vi "WiFi Receiver(FPGA).vi"() -> ()   [LabVIEW 2020]
doc: "Acquires data from the Rx ports and streams the data to the host while receiving data from the host and generating the resulting waveform at the Tx ports of the NI USRP 294x/295x device. Use this VI as a template for the Simple NI-USRP Streaming sample project."
uses:
  <instrlib>/_niInstr/Register Bus/v1/FPGA/Public/Read Cmd Data.ctl
  SubVIs/Stream Control State.ctl
  SubVIs/Rx Parameters 2945 2955.ctl
  Host/SubVIs/Start Trigger.ctl
  SubVIs/DDC Parameters 2945 2955.ctl
  <instrlib>/_niInstr/DSP/v1/Shared/Public/IQ Impairments.ctl
  <instrlib>/_niInstr/DSP/v1/Shared/Public/IQ Gain.ctl
  FPGA Bitfiles/Configuration Control.ctl
  <vilib>/Platform/TimedLoop/XDataNode/timing_clust.ctl
  <vilib>/Platform/TimedLoop/XDataNode/nitl_modes.ctl
  <vilib>/Platform/TimedLoop/XDataNode/wakeup.ctl
  SubVIs/Tx Parameters.ctl
  SubVIs/DUC Parameters.ctl
  <vilib>/rvi/Emulation/niFpgaSctlEmulationGetInTimedLoop.vi
  <vilib>/rvi/Emulation/niFpgaEmulationReportErrorSimple.vi
  <vilib>/rvi/Emulation/niFpgaGetClockAttributes.vi
  <vilib>/rvi/Emulation/niFpgaCriticalErrorInLSC.vi
  <vilib>/rvi/DataTransferAndStorage/Container/Common/niFpgaContainerExecOnDevCompGetState.vi
  <vilib>/rvi/Emulation/niFpgaEmulationIsFPGAContextNoSignature.vi
  <vilib>/rvi/errors/niFpgaSetErrorForExecOnDevCompSimple.vi
  <vilib>/rvi/eio/common/nirviEmuReportErrorAndStop.vi
  <vilib>/rvi/DataTransferAndStorage/Container/Common/niFpgaContainerGetUniqueNameForEmu.vi
  <vilib>/rvi/FIFO/Fifo_Resource/nirvififoEmulationSetSize.vi
  <vilib>/rvi/FIFO/Fifo_Resource/nirviFifoEmulationQueueMgr.vi
  <instcachedir>/0/nirviFifoEmulationQueueMgr_E5CAEC123FF24DC58D834DCA3CDAA9B5.lvgen/nirviFifoEmulationQueueMgr_E5CAEC123FF24DC58D834DCA3CDAA9B5_004.vi
  <vilib>/rvi/FIFO/Fifo_Resource/nirvififoEmulationDetermineInputValidOut.vi
  <vilib>/rvi/FIFO/Fifo_Resource/nirvififoEmulationCreateLock.vi
  <vilib>/rvi/Emulation/niFpgaProcessEmulError.vi
  <vilib>/rvi/FIFO/Fifo_Resource/nirvififoEmulationObtainLock.vi
  <vilib>/rvi/FIFO/Fifo_Resource/nirvififoEmulationReleaseLock.vi
  <vilib>/rvi/occurrence/nirviWaitOnOccurrenceBase.vi
  <vilib>/rvi/errors/nirviReportUnexpectedCaseInternalError.vi
  <vilib>/rvi/errors/nirviReportUnexpectedCaseInternalError (U32).vi
  <vilib>/Utility/error.llb/Clear Errors.vi
  <vilib>/rvi/interface/RandomDataEmulation/niFpgaRandomDataHandleErrors.vi
  <vilib>/Platform/TimedLoop/XDataNode/XDataNode.xnode
  <vilib>/rvi/DataTransferAndStorage/Container/XNode/niFpgaContainer.xnode
  <vilib>/rvi/FIFO/Fifo_Resource/niFpgaFifoEmulationRefIn.vi
  <vilib>/rvi/interface/RandomDataEmulation/nirviRandomDataFpgaReadWriteTemplate.vi
  <vilib>/Platform/TimedLoop/XDataNode/XDNodeRunTimeDep.lvlib
  <instrlib>/niUsrpRio/Config/v1/FPGA/niUsrpRio Config v1 FPGA.lvlib
  <instrlib>/_niInstr/DSP/v1/Shared/niInstr DSP v1 Shared.lvlib
  <instrlib>/_niInstr/Register Bus/v1/FPGA/niInstr Register Bus v1 FPGA.lvlib
panel:
  in  "use static frequency shift":bool
  in  "save before CFO":bool
  in  "before CFO compensation":bool
  in  "compensation":T1
  out "subcarrier index":fxp<+/-,9,9>
  out "channel estimate valid":bool=TRUE
  out "channel estimate":T2
  in  "configuration":T3={"primary channel selector"=0.0, "last OFDM symbol index"=0, "switch format detection states"=TRUE, "format"=enum."NON_HT_OFDM", "bandwidth"=enum."20MHz"}
  out "was packet detected true? 2":bool
  out "was packet start true?":bool
  in  "for filter":enum16{"20MHz", "40MHz"}(ring)
  in  "for shift":T4(ring)=enum."0MHz"
  out "packet start number":u32
  out "sample number":i16
  out "compensated CFO":fxp<+/-,48,0>
  out "packet detected":bool
  out "packet start":bool
  out "sample out valid":bool
  out "sample out":T5
  out "rx.parameters 2":T6={"rx.trigger select"=enum."Software", "rx.trigger enable"=FALSE, "rx.trigger sync enable"=FALSE, "rx.stream enable"=[FALSE, FALSE, FALSE, FALSE], "rx.software trigger"=FALSE, "rx.reset"=FALSE, "rx.abort"=FALSE, "rx.samples to acquire"=0, "rx.data sink"=enum."SFP Port 0", "rx.ddc parameters"=[{"output sample rate"=0.0, "delay"=0.0, "frequency shift"=0.0, "impairments"={"inline gain I"=0.0, "inline gain Q"=0.0, "cross gain I"=0.0, "cross gain Q"=0.0, "pre-gain offset I"=0.0, "pre-gain offset Q"=0.0, "post-gain offset I"=0.0, "post-gain offset Q"=0.0}, "phase"=0.0, "if frequency shift"=0.0}, {"output sample rate"=0.0, "delay"=0.0, "frequency shift"=0.0, "impairments"={"inline gain I"=0.0, "inline gain Q"=0.0, "cross gain I"=0.0, "cross gain Q"=0.0, "pre-gain offset I"=0.0, "pre-gain offset Q"=0.0, "post-gain offset I"=0.0, "post-gain offset Q"=0.0}, "phase"=0.0, "if frequency shift"=0.0}, {"output sample rate"=0.0, "delay"=0.0, "frequency shift"=0.0, "impairments"={"inline gain I"=0.0, "inline gain Q"=0.0, "cross gain I"=0.0, "cross gain Q"=0.0, "pre-gain offset I"=0.0, "pre-gain offset Q"=0.0, "post-gain offset I"=0.0, "post-gain offset Q"=0.0}, "phase"=0.0, "if frequency shift"=0.0}, {"output sample rate"=0.0, "delay"=0.0, "frequency shift"=0.0, "impairments"={"inline gain I"=0.0, "inline gain Q"=0.0, "cross gain I"=0.0, "cross gain Q"=0.0, "pre-gain offset I"=0.0, "pre-gain offset Q"=0.0, "post-gain offset I"=0.0, "post-gain offset Q"=0.0}, "phase"=0.0, "if frequency shift"=0.0}]} {"rx.ddc parameters"."if frequency shift" format="%#.48g"; "rx.ddc parameters"."frequency shift" format="%#.48g"}
  out "FIFO error out 2":errorcluster
  out "lol":bool
  in  "kek":bool
  in  "rx 3.if frequency shift":fxp<+/-,48,0> format="%#.48g"
  in  "rx 2.if frequency shift":fxp<+/-,48,0> format="%#.48g"
  in  "rx 1.if frequency shift":fxp<+/-,48,0> format="%#.48g"
  in  "rx 0.if frequency shift":fxp<+/-,48,0> format="%#.48g"
  in  "tx 1.led":enum16{"None", "RF 0/TX 1", "RF 1/TX 1"}(ring)
  in  "tx 0.led":enum16{"None", "RF 0/TX 1", "RF 1/TX 1"}(ring)
  in  "rx 0.led":T10(ring)
  in  "rx 1.led":T10(ring)
  in  "rx 2.led":T10(ring)
  in  "rx 3.led":T10(ring)
  in  "tx.data source":enum16{"SFP Port 0", "SFP Port 1", "Host"}(ring)=enum."Host"
  in  "tx.trigger sync enable":bool
  out "tx 1.number of iq data overflows":u64
  out "tx.dsp reset done":bool
  out "tx.state":T11
  out "tx 0.number of iq data overflows":u64
  out "tx.number of fifo underflows":u32
  out "tx.samples processed":u32
  in  "tx.trigger enable":bool
  in  "tx.software trigger":bool
  in  "tx.trigger select":T7=enum."Immediate"
  in  "tx 1.stream enable":bool
  in  "tx 0.stream enable":bool
  in  "tx.samples to generate":u32
  in  "tx.reset":bool=TRUE
  in  "tx.abort":bool
  in  "tx 1.gain":T12={"gain I"=1.0, "gain Q"=1.0}
  in  "tx 1.phase":fxp<+/-,21,0>
  in  "tx 1.frequency shift":fxp<+/-,48,0> format="%#.48g"
  in  "tx 1.impairments":T9={"inline gain I"=0.9999923706054688, "inline gain Q"=0.9999923706054688, "cross gain I"=0.0, "cross gain Q"=0.0, "pre-gain offset I"=0.0, "pre-gain offset Q"=0.0, "post-gain offset I"=0.0, "post-gain offset Q"=0.0}
  in  "tx 0.gain":T12={"gain I"=1.0, "gain Q"=1.0}
  in  "tx 0.impairments":T9={"inline gain I"=0.9999923706054688, "inline gain Q"=0.9999923706054688, "cross gain I"=0.0, "cross gain Q"=0.0, "pre-gain offset I"=0.0, "pre-gain offset Q"=0.0, "post-gain offset I"=0.0, "post-gain offset Q"=0.0}
  in  "tx 0.phase":fxp<+/-,21,0>
  in  "tx 0.frequency shift":fxp<+/-,48,0> format="%#.48g"
  in  "tx.delay":fxp<+/-,18,0>
  in  "tx.input sample rate":fxp<+,48,1>
  out "rx.status":T13={"rx.state"=enum."Idle", "rx.samples processed"=0, "rx.number of fifo overflows"=0, "rx.number of iq data overflows"=[0, 0, 0, 0], "rx.dsp reset done"=FALSE}
  in  "rx 2.stream enable":bool
  in  "rx 3.stream enable":bool
  out "rx 3.number of iq data overflows":u64
  out "rx 2.number of iq data overflows":u64
  in  "rx 3.impairments":T9={"inline gain I"=0.9999923706054688, "inline gain Q"=0.9999923706054688, "cross gain I"=0.0, "cross gain Q"=0.0, "pre-gain offset I"=0.0, "pre-gain offset Q"=0.0, "post-gain offset I"=0.0, "post-gain offset Q"=0.0}
  in  "rx 3.frequency shift":fxp<+/-,48,0> format="%#.48g"
  in  "rx 3.phase":fxp<+/-,21,0>
  in  "rx 2.impairments":T9={"inline gain I"=0.9999923706054688, "inline gain Q"=0.9999923706054688, "cross gain I"=0.0, "cross gain Q"=0.0, "pre-gain offset I"=0.0, "pre-gain offset Q"=0.0, "post-gain offset I"=0.0, "post-gain offset Q"=0.0}
  in  "rx 2.frequency shift":fxp<+/-,48,0> format="%#.48g"
  in  "rx 2.phase":fxp<+/-,21,0>
  in  "RF 1/Tx/Enable":bool
  in  "RF 1/Rx/Enable":bool
  in  "RF 0/Tx/Enable":bool
  in  "RF 0/Rx/Enable":bool
  in  "rx.output sample rate":fxp<+,48,1>
  in  "rx.delay":fxp<+/-,16,0>
  in  "rx 0.frequency shift":fxp<+/-,48,0> format="%#.48g"
  in  "rx 0.phase":fxp<+/-,21,0>
  in  "rx 0.impairments":T9={"inline gain I"=0.9999923706054688, "inline gain Q"=0.9999923706054688, "cross gain I"=0.0, "cross gain Q"=0.0, "pre-gain offset I"=0.0, "pre-gain offset Q"=0.0, "post-gain offset I"=0.0, "post-gain offset Q"=0.0}
  in  "rx 1.impairments":T9={"inline gain I"=0.9999923706054688, "inline gain Q"=0.9999923706054688, "cross gain I"=0.0, "cross gain Q"=0.0, "pre-gain offset I"=0.0, "pre-gain offset Q"=0.0, "post-gain offset I"=0.0, "post-gain offset Q"=0.0}
  in  "rx 1.frequency shift":fxp<+/-,48,0> format="%#.48g"
  in  "rx 1.phase":fxp<+/-,21,0>
  in  "rx.reset":bool=TRUE
  in  "rx.samples to acquire":u32
  in  "rx.abort":bool
  in  "rx 0.stream enable":bool
  in  "rx 1.stream enable":bool
  in  "rx.trigger select":T7=enum."Immediate"
  in  "rx.software trigger":bool
  in  "rx.trigger enable":bool
  out "rx.parameters":T6={"rx.trigger select"=enum."Software", "rx.trigger enable"=FALSE, "rx.trigger sync enable"=FALSE, "rx.stream enable"=[FALSE, FALSE, FALSE, FALSE], "rx.software trigger"=FALSE, "rx.reset"=FALSE, "rx.abort"=FALSE, "rx.samples to acquire"=0, "rx.data sink"=enum."SFP Port 0", "rx.ddc parameters"=[{"output sample rate"=0.0, "delay"=0.0, "frequency shift"=0.0, "impairments"={"inline gain I"=0.0, "inline gain Q"=0.0, "cross gain I"=0.0, "cross gain Q"=0.0, "pre-gain offset I"=0.0, "pre-gain offset Q"=0.0, "post-gain offset I"=0.0, "post-gain offset Q"=0.0}, "phase"=0.0, "if frequency shift"=0.0}, {"output sample rate"=0.0, "delay"=0.0, "frequency shift"=0.0, "impairments"={"inline gain I"=0.0, "inline gain Q"=0.0, "cross gain I"=0.0, "cross gain Q"=0.0, "pre-gain offset I"=0.0, "pre-gain offset Q"=0.0, "post-gain offset I"=0.0, "post-gain offset Q"=0.0}, "phase"=0.0, "if frequency shift"=0.0}, {"output sample rate"=0.0, "delay"=0.0, "frequency shift"=0.0, "impairments"={"inline gain I"=0.0, "inline gain Q"=0.0, "cross gain I"=0.0, "cross gain Q"=0.0, "pre-gain offset I"=0.0, "pre-gain offset Q"=0.0, "post-gain offset I"=0.0, "post-gain offset Q"=0.0}, "phase"=0.0, "if frequency shift"=0.0}, {"output sample rate"=0.0, "delay"=0.0, "frequency shift"=0.0, "impairments"={"inline gain I"=0.0, "inline gain Q"=0.0, "cross gain I"=0.0, "cross gain Q"=0.0, "pre-gain offset I"=0.0, "pre-gain offset Q"=0.0, "post-gain offset I"=0.0, "post-gain offset Q"=0.0}, "phase"=0.0, "if frequency shift"=0.0}]} {"rx.ddc parameters"."if frequency shift" format="%#.48g"; "rx.ddc parameters"."frequency shift" format="%#.48g"}
  out "rx.samples processed":u32
  out "rx.state":T11
  out "rx 0.number of iq data overflows":u64
  out "rx.number of fifo overflows":u32
  out "rx.dsp reset done":bool
  out "rx 1.number of iq data overflows":u64
  in  "rx.trigger sync enable":bool
  in  "rx.data sink":enum16{"SFP Port 0", "SFP Port 1", "Host"}(ring)=enum."Host"
  in  "reg.host read.go rcvd 0":bool
  out "reg.notify host.go 0":bool
  in  "reg.notify host.go rcvd 0":bool
  out "reg.host read.data 0":T14
  in  "reg.reset 0":bool
  # "USRP RIO MuSiC Localization FPGA"
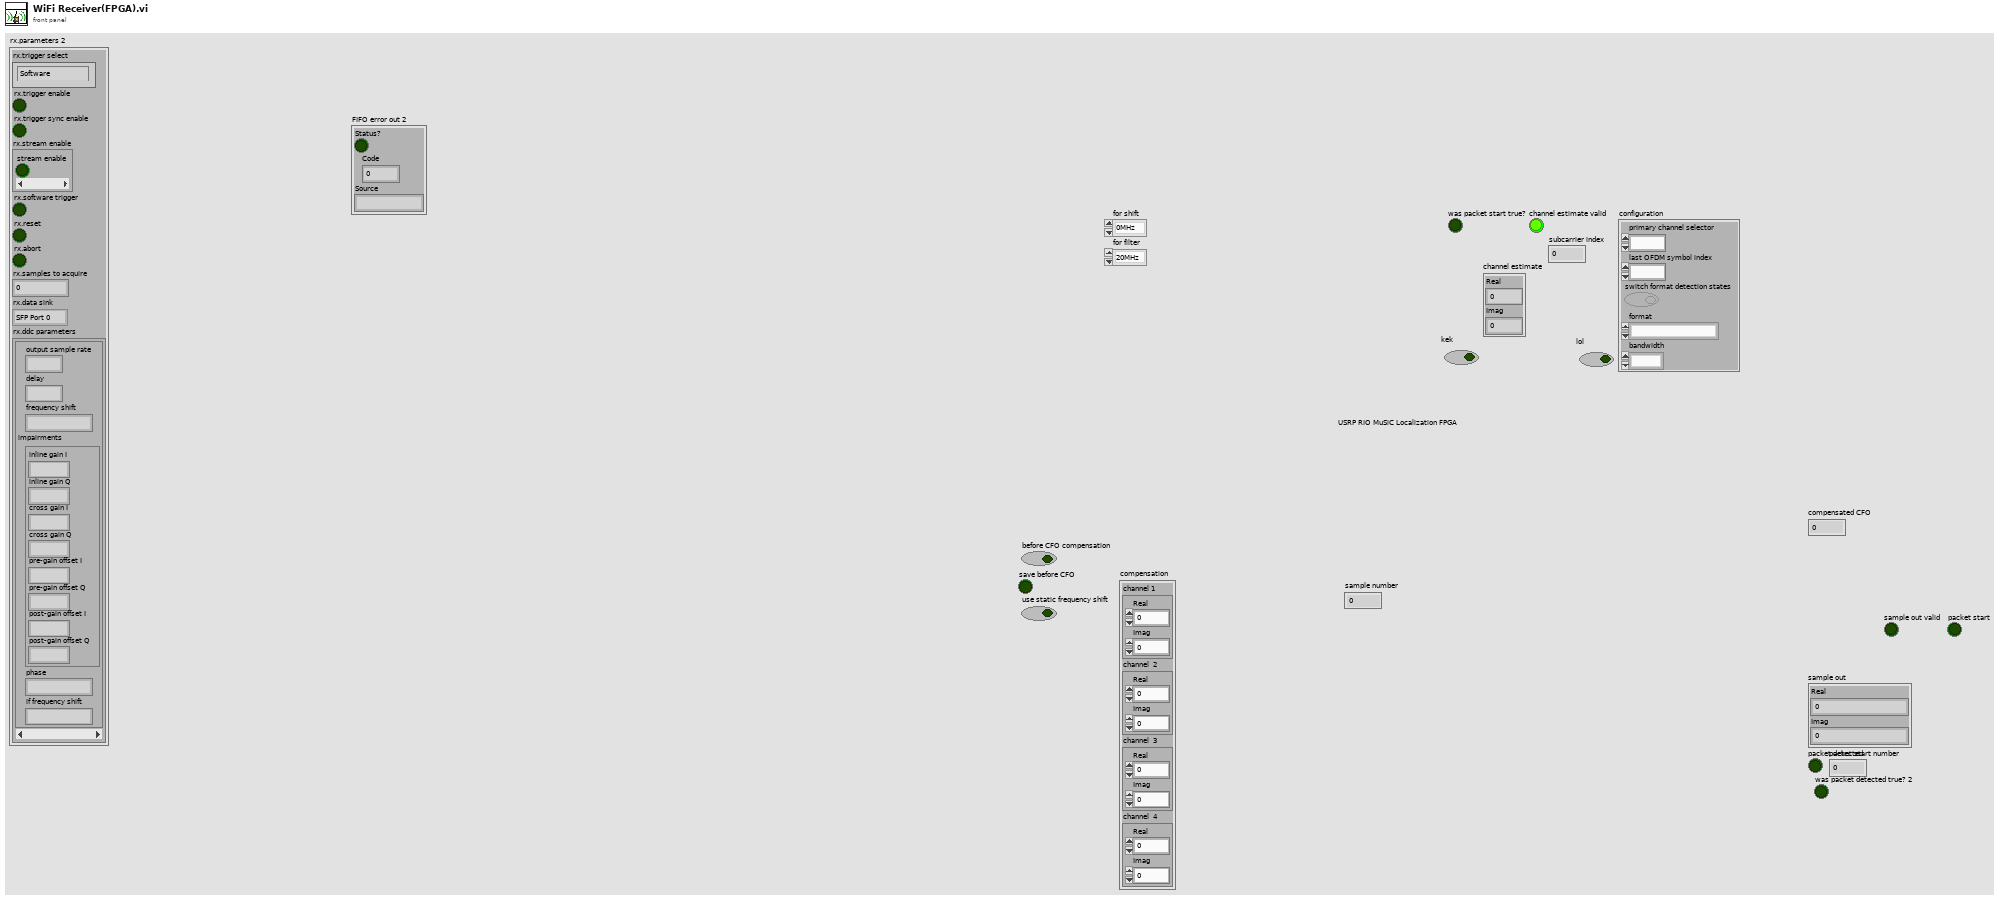
[diagram p1: front panel]
types:
  T1 = cluster{"channel 1 ":cluster{"Real":fxp<+/-,16,3>, "Imag":fxp<+/-,16,3>}, "channel  2":cluster{"Real":fxp<+/-,16,3>, "Imag":fxp<+/-,16,3>}, "channel  3":cluster{"Real":fxp<+/-,16,3>, "Imag":fxp<+/-,16,3>}, "channel  4":cluster{"Real":fxp<+/-,16,3>, "Imag":fxp<+/-,16,3>}}
  T2 = cluster{"Real":fxp<+/-,25,4>, "Imag":fxp<+/-,25,4>}
  T3 = typedef "Configuration Control.ctl" = cluster{"primary channel selector":fxp<+,2,0>, "last OFDM symbol index":u16, "switch format detection states":bool, "format":enum16{"NON_HT_OFDM", "VHT", "NON_HT_DUP_OFDM"}, "bandwidth":enum16{"20MHz", "40MHz", "80MHz"}}
  T4 = enum16{"-30MHz", "-20MHz", "-10MHz", "0MHz", "10MHz", "20MHz", "30MHz"}
  T5 = cluster{"Real":fxp<+/-,16,3>, "Imag":fxp<+/-,16,3>}
  T6 = typedef "Rx Parameters 2945 2955.ctl" = cluster{"rx.trigger select":T7, "rx.trigger enable":bool, "rx.trigger sync enable":bool, "rx.stream enable":bool[], "rx.software trigger":bool, "rx.reset":bool, "rx.abort":bool, "rx.samples to acquire":u32, "rx.data sink":enum16{"SFP Port 0", "SFP Port 1", "Host"}, "rx.ddc parameters":T8[]}
  T7 = typedef "Start Trigger.ctl" = enum8{"Software", "Digital Edge", "Rx Start Trigger", "Tx Start Trigger", "Immediate", "Future Time Event"}
  T8 = typedef "DDC Parameters 2945 2955.ctl" = cluster{"output sample rate":fxp<+,48,1>, "delay":fxp<+/-,16,0>, "frequency shift":fxp<+/-,48,0>, "impairments":T9, "phase":fxp<+/-,21,0>, "if frequency shift":fxp<+/-,48,0>}
  T9 = typedef "niInstr DSP v1 Shared.lvlib/IQ Impairments.ctl" = cluster{"inline gain I":fxp<+/-,18,1>, "inline gain Q":fxp<+/-,18,1>, "cross gain I":fxp<+/-,18,1>, "cross gain Q":fxp<+/-,18,1>, "pre-gain offset I":fxp<+/-,18,1>, "pre-gain offset Q":fxp<+/-,18,1>, "post-gain offset I":fxp<+/-,18,1>, "post-gain offset Q":fxp<+/-,18,1>}
  T10 = enum16{"None", "RF 0/RX 1", "RF 0/RX 2", "RF 1/RX 1", "RF 1/RX 2"}
  T11 = typedef "Stream Control State.ctl" = enum16{"Idle", "Active"}
  T12 = typedef "niInstr DSP v1 Shared.lvlib/IQ Gain.ctl" = cluster{"gain I":fxp<+/-,24,3>, "gain Q":fxp<+/-,24,3>}
  T13 = cluster{"rx.state":T11, "rx.samples processed":u32, "rx.number of fifo overflows":u32, "rx.number of iq data overflows":u64[], "rx.dsp reset done":bool}
  T14 = typedef "niInstr Register Bus v1 FPGA.lvlib/Read Cmd Data.ctl" = cluster{"go":bool, "data":u32}
  T15 = typedef "XDNodeRunTimeDep.lvlib/timing_clust.ctl" = cluster{"Expected End [f-1]":u64, "Actual End [f-1]":u64, "Finished Late? [f-1]":bool, "Expected End [i-1]":u64, "Actual End [i-1]":u64, "Finished Late? [i-1]":bool, "Expected Start [i]":u64, "Actual Start [i]":u64, "Expected Start [f]":u64, "Actual Start [f]":u64, "Source Name":string, "Structure Name":string, "Period":i64, "Deadline":i64, "Offset":i64, "Start":i64, "Priority":i32, "Timeout":i32, "Mode":T16, "Wakeup Reason":T17, "Error":errorcluster, "Source Type":string, "Secondary Source Type":string, "Global End Time":u64, "Global Start Time":u64, "Frame Duration":u64, "Iteration Duration":u64, "Assigned CPU":i32, "I/O Scan Engine Mode":u32}
  T16 = typedef "XDNodeRunTimeDep.lvlib/nitl_modes.ctl" = enum32{"No Change", "Process missed periods, maintain original phase", "Discard missed periods, maintain original phase", "Process missed periods, ignore original phase", "Discard missed periods, ignore original phase"}
  T17 = typedef "XDNodeRunTimeDep.lvlib/wakeup.ctl" = enum32{"Normal", "Aborted", "Asynchronous wakeup", "Timing source error", "Timed loop error", "Timeout"}
  T18 = cluster{"rx 0.led":enum16{"None", "RF 0/RX 1", "RF 0/RX 2", "RF 1/RX 1", "RF 1/RX 2"}, "rx 1.led":enum16{"None", "RF 0/RX 1", "RF 0/RX 2", "RF 1/RX 1", "RF 1/RX 2"}, "rx 2.led":enum16{"None", "RF 0/RX 1", "RF 0/RX 2", "RF 1/RX 1", "RF 1/RX 2"}, "rx 3.led":enum16{"None", "RF 0/RX 1", "RF 0/RX 2", "RF 1/RX 1", "RF 1/RX 2"}}
  T19 = cluster{"rx.trigger select":T7, "rx.trigger enable":bool, "rx.trigger sync enable":bool, bool[], "rx.software trigger":bool, "rx.reset":bool, "rx.abort":bool, "rx.samples to acquire":u32, "rx.data sink":enum16{"SFP Port 0", "SFP Port 1", "Host"}, T8[]}
  T20 = cluster{"DAC FIFO Reset":refnum<k21>, "RF 0 Rx Swap IQ":refnum<k21>, "RF 0 Rx Negate I":refnum<k21>, "RF 0 Rx Negate Q":refnum<k21>, "RF 0 Rx Data Valid":refnum<k21>, "RF 0 Rx Data Ever Invalid":refnum<k21>, "clear RF 0 Rx Data Ever Invalid":refnum<k21>, "RF 0 Tx Swap IQ":refnum<k21>, "RF 0 Tx Negate I":refnum<k21>, "RF 0 Tx Negate Q":refnum<k21>, "RF 1 Rx Swap IQ":refnum<k21>, "RF 1 Rx Negate I":refnum<k21>, "RF 1 Rx Negate Q":refnum<k21>, "RF 1 Rx Data Valid":refnum<k21>, "RF 1 Rx Data Ever Invalid":refnum<k21>, "clear RF 1 Rx Data Ever Invalid":refnum<k21>, "RF 1 Tx Swap IQ":refnum<k21>, "RF 1 Tx Negate I":refnum<k21>, "RF 1 Tx Negate Q":refnum<k21>}
  T21 = typedef "niUsrpRio Synchronization v1 FPGA.lvlib/Resources.ctl" = cluster{"master":refnum<k21>, "meas.enable":refnum<k21>, "meas.ready":refnum<k21>, "meas.reset":refnum<k21>, "meas.arm":refnum<k21>, "meas.valid":refnum<k21>, "meas.value":refnum<k21>, "meas.oversample factor":refnum<k21>, "cptr":refnum<k21>, "cptr.adjust":refnum<k21>, "cptr.period":refnum<k21>}
  T22 = typedef "niUsrpRio Time v1 FPGA.lvlib/Time Resources.ctl" = cluster{"reset":refnum<k21>, "time":refnum<k21>, "time.previous cptr":refnum<k21>, "new time":refnum<k21>, "new time.when":refnum<k21>, "new time.set":refnum<k21>, "which edge of ref":refnum<k21>, "pps source":refnum<k21>, "internal pps period":refnum<k21>}
  T23 = typedef "niUsrpRio Time v1 FPGA.lvlib/Future Event Resources.ctl" = cluster{"reset":refnum<k21>, "future event.time":refnum<k21>, "future event.ready":refnum<k21>, "future event.set":refnum<k21>, "future event.clear":refnum<k21>, "future event.set in past":refnum<k21>}
  T24 = cluster{"time.resources":T22, "future event.resources":T23, "future event.resources":T23, "future event.resources":T23}
  T25 = typedef "Clock Cross Resources.ctl" = cluster{"register instruction":refnum<k21>, "read completion":refnum<k21>}
  T26 = typedef "niInstr Register Bus v1 FPGA.lvlib/Register Instruction.ctl" = cluster{"subsystem":u8, "address":u16, "data":u32, "valid":bool, "read":bool}
  T27 = typedef "niInstr Register Bus v1 FPGA.lvlib/Read Completion.ctl" = cluster{"data":u32, "valid":bool}
  T28 = typedef "Tx Parameters.ctl" = cluster{"tx.trigger select":T7, "tx.trigger enable":bool, "tx.trigger sync enable":bool, "tx.stream enable":bool[], "tx.software trigger":bool, "tx.reset":bool, "tx.abort":bool, "tx.samples to generate":u32, "tx.data source":enum16{"SFP Port 0", "SFP Port 1", "Host"}, "tx.duc parameters":T29[]}
  T29 = typedef "DUC Parameters.ctl" = cluster{"frequency shift":fxp<+/-,48,0>, "impairments":T9, "phase":fxp<+/-,21,0>, "input sample rate":fxp<+,48,1>, "gain":T12, "delay":fxp<+/-,18,0>}
  T30 = cluster{"subcarrier index":u8, "OFDM symbol index":u16, "frequency offset index":fxp<+/-,9,9>, "OFDM symbol start":bool, "valid":bool}
  T31 = cluster{"subcarrier channel":cluster{"Real":fxp<+/-,25,4>, "Imag":fxp<+/-,25,4>}, "subcarrier channel 2":cluster{"Real":fxp<+/-,25,4>, "Imag":fxp<+/-,25,4>}, "subcarrier channel 3":cluster{"Real":fxp<+/-,25,4>, "Imag":fxp<+/-,25,4>}, "subcarrier channel 4":cluster{"Real":fxp<+/-,25,4>, "Imag":fxp<+/-,25,4>}}
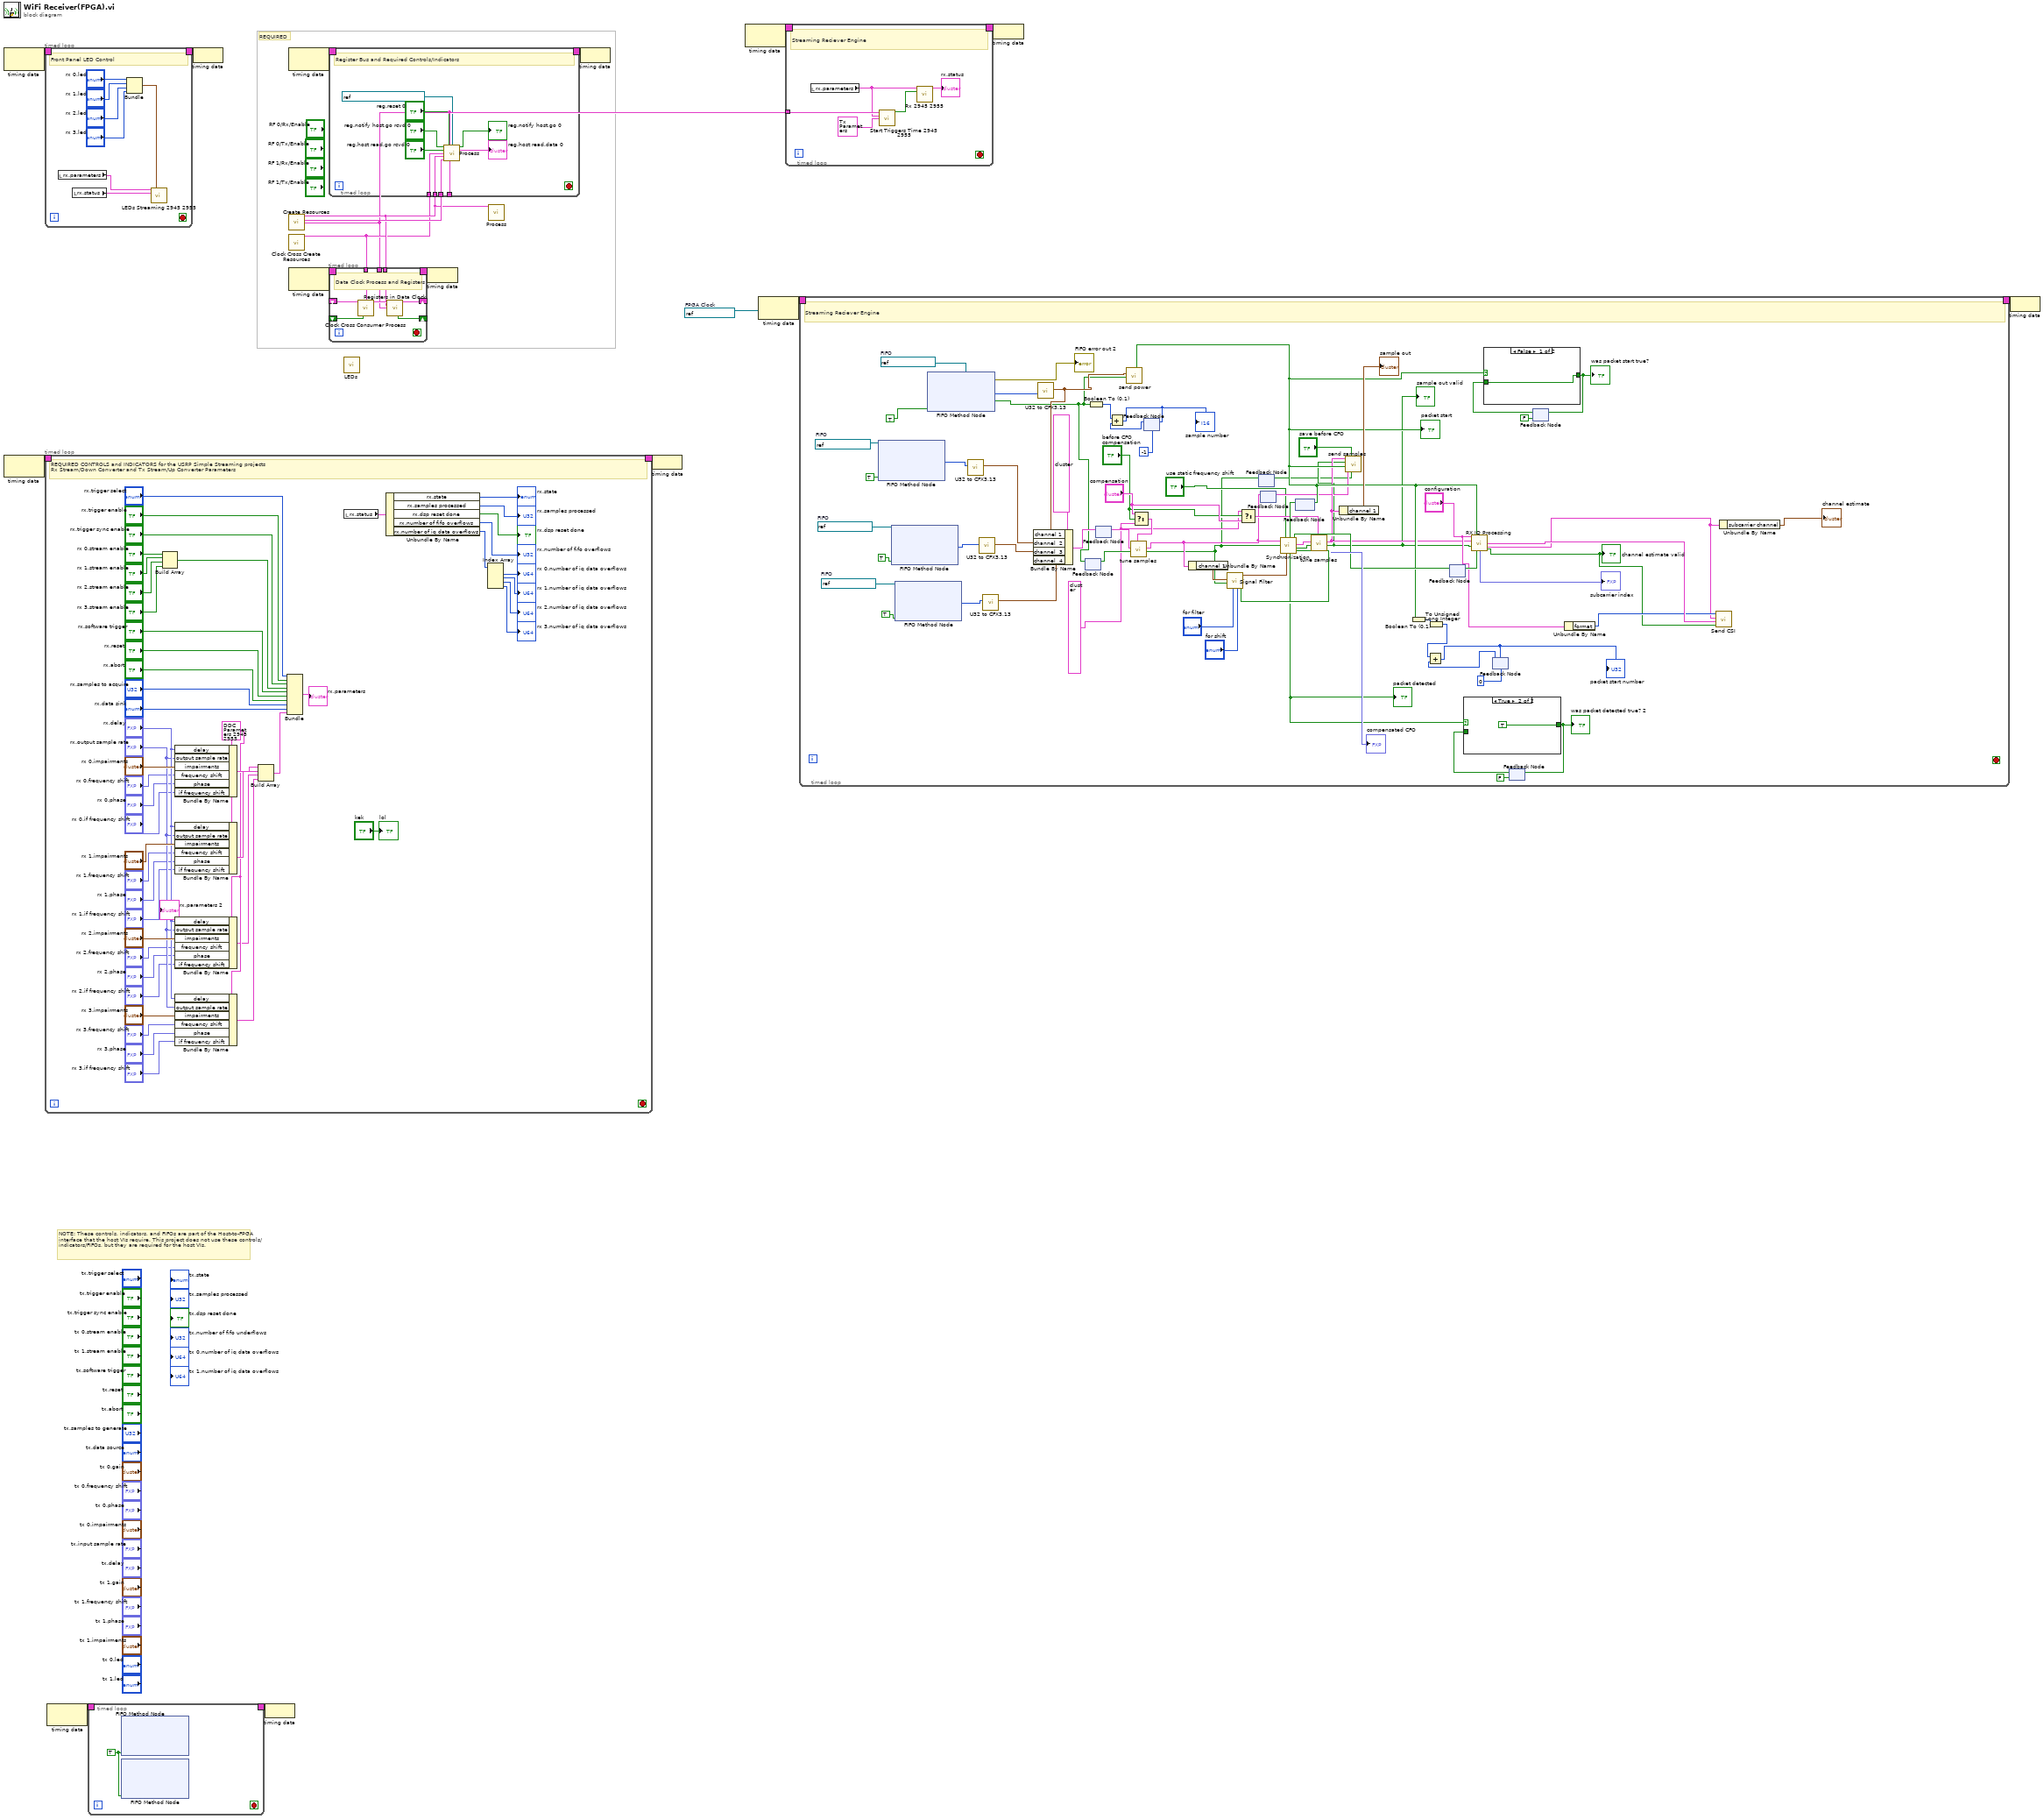
[diagram p0: block diagram]
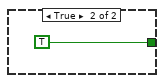
[diagram p3: hidden frame]
diagram:
  w1 = refnum<k21> "PHY 250MHz"  # FPGA Clock
  # "NOTE: These controls, indicators, and FIFOs are part of the Host-to-FPGA interface that the host VIs require. This project does not use these controls/indicators/FIFOs, but they are required for the host VIs."
  # "REQUIRED"
  n1 = node-c288() -> (w5:T15)  [unwired: 1 in]
  n2 = node-c288() -> (w15:T15)  [unwired: 1 in]
  n3 = timed-loop {
    timing: w5 -> [_]
    timing-out: [_] -> w4
    stop <- _ stop-if-true
    # "Front Panel LED Control"
    n4 = local read "rx.parameters"() -> (w21:T6)
    n5 = local read "rx.status"() -> (w20:T13)
    n6 = Bundle("rx 0.led"="rx 0.led", "rx 1.led"="rx 1.led", "rx 2.led"="rx 2.led", "rx 3.led"="rx 3.led") -> (w22:T18)  [unwired: 1 in]
    n7 = call "LEDs Streaming 2945 2955.vi"("rx.parameters"=w21, "rx.leds"=w22, "rx.status"=w20) -> ()  [unwired: 13 in]
  }
  n8 = timed-loop {
    timing: w15 -> [_]
    timing-out: [_] -> w14
    stop <- _ stop-if-true
    w60 = T8 {"output sample rate"=1.0, "delay"=0.0, "frequency shift"=0.0, "impairments"={"inline gain I"=0.9999923706054688, "inline gain Q"=0.9999923706054688, "cross gain I"=0.0, "cross gain Q"=0.0, "pre-gain offset I"=0.0, "pre-gain offset Q"=0.0, "post-gain offset I"=0.0, "post-gain offset Q"=0.0}, "phase"=0.0, "if frequency shift"=0.0} ("DDC Parameters")
    # "REQUIRED CONTROLS and INDICATORS for the USRP Simple Streaming projects\nRx Stream/Down Converter and Tx Stream/Up Converter Parameters"
    n9 = Build Array("rx 0.stream enable", "rx 1.stream enable", "rx 2.stream enable", "rx 3.stream enable") -> (w41:bool[])
    n10 = Bundle By Name(cluster=w60, "delay"="rx.delay", "output sample rate"="rx.output sample rate", "impairments"="rx 0.impairments", "frequency shift"="rx 0.frequency shift", "phase"="rx 0.phase", "if frequency shift"="rx 0.if frequency shift") -> (w76:T8)
    n11 = Bundle By Name(cluster=w60, "delay"="rx.delay", "output sample rate"="rx.output sample rate", "impairments"="rx 1.impairments", "frequency shift"="rx 1.frequency shift", "phase"="rx 1.phase", "if frequency shift"="rx 1.if frequency shift") -> (w77:T8)
    n12 = Bundle By Name(cluster=w60, "delay"="rx.delay", "output sample rate"="rx.output sample rate", "impairments"="rx 2.impairments", "frequency shift"="rx 2.frequency shift", "phase"="rx 2.phase", "if frequency shift"="rx 2.if frequency shift") -> (w57:T8)
    n13 = Bundle By Name(cluster=w60, "delay"="rx.delay", "output sample rate"="rx.output sample rate", "impairments"="rx 3.impairments", "frequency shift"="rx 3.frequency shift", "phase"="rx 3.phase", "if frequency shift"="rx 3.if frequency shift") -> (w56:T8)
    n14 = Build Array(w76, w77, w57, w56) -> (w67:T8[])
    n15 = Bundle("rx.trigger select"="rx.trigger select", "rx.trigger enable"="rx.trigger enable", "rx.trigger sync enable"="rx.trigger sync enable", w41, "rx.software trigger"="rx.software trigger", "rx.reset"="rx.reset", "rx.abort"="rx.abort", "rx.samples to acquire"="rx.samples to acquire", "rx.data sink"="rx.data sink", w67) -> (→"rx.parameters":T19)  [unwired: 1 in]
    n16 = local read "rx.status"() -> (w66:T13)
    n17 = Unbundle By Name(w66) -> ("rx.state"=→"rx.state":T11, "rx.samples processed"=→"rx.samples processed":u32, "rx.dsp reset done"=→"rx.dsp reset done":bool, "rx.number of fifo overflows"=→"rx.number of fifo overflows":u32, "rx.number of iq data overflows"=w38:u64[])
    n18 = Index Array(array=w38) -> (element #1=→"rx 0.number of iq data overflows":u64, element #2=→"rx 1.number of iq data overflows":u64, element #3=→"rx 2.number of iq data overflows":u64, element #4=→"rx 3.number of iq data overflows":u64)  [unwired: 4 in]
    "lol" <- "kek"
  }
  n19 = node-c288() -> (w7:T15)  [unwired: 1 in]
  n20 = timed-loop {
    timing: w7 -> [_]
    timing-out: [_] -> w6
    stop <- _ stop-if-true
    w80 = TRUE ("Ready for Output")
    n21 = xnode ("FIFO Method Node")("Ready for Output"=w80) -> ()  [unwired: 1 in, 3 out]
    n22 = xnode ("FIFO Method Node")("Ready for Output"=w80) -> ()  [unwired: 1 in, 3 out]
  }
  n23 = node-c288(w4) -> ()
  n24 = node-c288(w6) -> ()
  n25 = node-c288() -> (w19:T15)  [unwired: 1 in]
  n26 = call "Create Resources.vi"() -> ("config.resources"=w10:T20, "sync.resources"=w13:T21, "time.resources"=w8:T24)  [unwired: 13 in]
  n27 = call "Clock Cross Create Resources.vi"() -> ("resources"=w9:T25)  [unwired: 15 in]
  n28 = node-c288() -> (w12:T15)  [unwired: 1 in]
  n29 = timed-loop "Register Bus and Required Controls/Indicators" {
    timing: w19 -> [_]
    timing-out: [_] -> w18
    tunnel: w10 -> [w85]
    tunnel: w13 -> [w84]
    tunnel: w8 -> [w83]
    tunnel: w9 -> [w86]
    stop <- _ stop-if-true
    # "Register Bus and Required Controls/Indicators"
    n30 = call <instrlib>:"Process.vi"("reg.notify host.go rcvd"="reg.notify host.go rcvd 0", "reg.reset"="reg.reset 0", "reg.instruction fifo"=refnum<k21> "reg.host instruction fifo 0" ("reg.host instruction fifo"), "reg.host read.go rcvd"="reg.host read.go rcvd 0", "clock cross resources"=w86, "config.resources"=w85, "sync.resources"=w84, "time.resources"=w83) -> ("reg.notify host.go"=→"reg.notify host.go 0":bool, "reg.host read.data"=→"reg.host read.data 0":T14)  [unwired: 6 in]
  }
  n31 = timed-loop {
    timing: w12 -> [_]
    timing-out: [_] -> w11
    shift-right: [w101] -> _
    shift-left: _ -> [w98]
    shift-right: [w100] -> _
    shift-left: _ -> [w99]
    tunnel: w10 -> [w97]
    tunnel: w9 -> [w96]
    tunnel: w8 -> [w95]
    stop <- _ stop-if-true
    # "Data Clock Process and Registers"
    n32 = call "Clock Cross Consumer Process.vi"("read completion"=w98, "resources"=w96, "ready for output"=w99) -> ("register instruction"=w102:T26)  [unwired: 12 in]
    n33 = call "Registers in Data Clock.vi"("register instruction"=w102, "config.resources"=w97, "time.resources"=w95) -> ("read completion out"=w101:T27, "ready for input"=w100:bool)  [unwired: 11 in]
  }
  n34 = call "LEDs.vi"() -> ()  [unwired: 1 in]
  n35 = node-c288(w11) -> ()
  n36 = call <instrlib>:"Process.vi"("resources"=w10) -> ()  [unwired: 15 in]
  n37 = node-c288(w18) -> ()
  n38 = node-c288(w14) -> ()
  n39 = node-c288() -> (w17:T15)  [unwired: 1 in]
  n40 = node-c288(w1) -> (w3:T15)
  n41 = timed-loop "Streaming Transceiver Engine" {
    timing: w17 -> [_]
    timing-out: [_] -> w16
    tunnel: w8 -> [w108]
    stop <- _ stop-if-true
    # "Streaming Reciever Engine"
    n42 = local read "rx.parameters"() -> (w107:T6)
    n43 = call "Start Triggers Time 2945 2955.vi"("time.resources"=w108, "rx.parameters"=w107, "tx.parameters"=T28 {"tx.trigger select"=enum."Software", "tx.trigger enable"=FALSE, "tx.trigger sync enable"=FALSE, "tx.stream enable"=[FALSE, FALSE], "tx.software trigger"=FALSE, "tx.reset"=FALSE, "tx.abort"=FALSE, "tx.samples to generate"=0, "tx.data source"=enum."SFP Port 0", "tx.duc parameters"=[{"frequency shift"=0.0, "impairments"={"inline gain I"=0.0, "inline gain Q"=0.0, "cross gain I"=0.0, "cross gain Q"=0.0, "pre-gain offset I"=0.0, "pre-gain offset Q"=0.0, "post-gain offset I"=0.0, "post-gain offset Q"=0.0}, "phase"=0.0, "input sample rate"=0.0, "gain"={"gain I"=0.0, "gain Q"=0.0}, "delay"=0.0}, {"frequency shift"=0.0, "impairments"={"inline gain I"=0.0, "inline gain Q"=0.0, "cross gain I"=0.0, "cross gain Q"=0.0, "pre-gain offset I"=0.0, "pre-gain offset Q"=0.0, "post-gain offset I"=0.0, "post-gain offset Q"=0.0}, "phase"=0.0, "input sample rate"=0.0, "gain"={"gain I"=0.0, "gain Q"=0.0}, "delay"=0.0}]}) -> ("rx.start trigger"=w109:bool)  [unwired: 11 in, 1 out]
    n44 = call "Rx 2945 2955.vi"("rx.parameters"=w107, "rx.start trigger"=w109) -> ("rx.status"=→"rx.status":T13)  [unwired: 13 in]
  }
  n45 = timed-loop "Streaming Transceiver Engine" {
    timing: w3 -> [_]
    timing-out: [_] -> w2
    stop <- _ stop-if-true
    w114 = T1 {"channel 1 "={"Real"=1.0, "Imag"=0.0}, "channel  2"={"Real"=1.0, "Imag"=0.0}, "channel  3"={"Real"=1.0, "Imag"=0.0}, "channel  4"={"Real"=1.0, "Imag"=0.0}} ("f")
    w165 = refnum<k21> "RF to RX FIFO 3"  # FIFO
    w167 = refnum<k21> "RF to RX FIFO 2"  # FIFO
    w169 = refnum<k21> "RF to RX FIFO 1"  # FIFO
    w181 = refnum<k21> "RF to RX FIFO 0"  # FIFO
    # "Streaming Reciever Engine"
    n46 = xnode ("FIFO Method Node")("Ready for Output"=TRUE, "FIFO In"=w169) -> ("Element"=w144:u32)  [unwired: 1 in, 3 out]
    n47 = xnode ("FIFO Method Node")("Ready for Output"=TRUE, "FIFO In"=w167) -> ("Element"=w143:u32)  [unwired: 1 in, 3 out]
    n48 = xnode ("FIFO Method Node")("Ready for Output"=TRUE, "FIFO In"=w165) -> ("Element"=w142:u32)  [unwired: 1 in, 3 out]
    n49 = xnode ("FIFO Method Node")("Ready for Output"=TRUE, "FIFO In"=w181) -> ("Element"=w172:u32, "Output Valid"=w118:bool, "error out"=→"FIFO error out 2":errorcluster)  [unwired: 1 in, 1 out]
    n50 = call "U32 to CFX3.13.vi"("Data in"=w144) -> ("Data out"=w140:T5)  [unwired: 10 in]
    n51 = call "U32 to CFX3.13.vi"("Data in"=w143) -> ("Data out"=w139:T5)  [unwired: 10 in]
    n52 = call "U32 to CFX3.13.vi"("Data in"=w142) -> ("Data out"=w138:T5)  [unwired: 10 in]
    n53 = call "U32 to CFX3.13.vi"("Data in"=w172) -> ("Data out"=w134:T5)  [unwired: 10 in]
    n54 = Bundle By Name(cluster=T1 {"channel 1 "={"Real"=0.0, "Imag"=0.0}, "channel  2"={"Real"=0.0, "Imag"=0.0}, "channel  3"={"Real"=0.0, "Imag"=0.0}, "channel  4"={"Real"=0.0, "Imag"=0.0}}, "channel 1"=w134, "channel  2"=w140, "channel  3"=w139, "channel  4"=w138) -> (w120:T1)
    n55 = feedback #1() -> (w117:bool)  [unwired: 1 in]
    n56 = feedback-in #1(w118) -> ()
    n57 = Boolean To (0,1)(Boolean=w118) -> (0, 1=w176:i16)
    n58 = feedback #2() -> (w119:T1)  [unwired: 1 in]
    n59 = feedback-in #2(w120) -> ()
    n60 = Select(t="compensation", s="before CFO compensation", f=w114) -> (s? t:f=w127:T1)
    n61 = call "tune samples.vi"("compensation"=w127, "input valid"=w117, "channels in"=w119) -> ("output valid"=w112:bool, "channels out"=w121:T1)  [unwired: 7 in]
    n62 = feedback #3(i16 -1) -> (w174:i16)
    n63 = Add(x=w176, y=w174) -> (x+y=w173:i16)
    "sample number" <- w173
    n64 = feedback-in #3(w173) -> ()
    n65 = Unbundle By Name(w121) -> ("channel 1"=w122:T5)
    n66 = call "Signal Filter.vi"("for shift"="for shift", "for filter"="for filter", "input valid"=w112, "sample in"=w122) -> ("output valid"=w179:bool, "primary channel sample"=w178:T5)  [unwired: 6 in]
    n67 = Select(t=w114, s="before CFO compensation", f="compensation") -> (s? t:f=w126:T1)
    n68 = feedback #4() -> (w113:bool)  [unwired: 1 in]
    n69 = feedback-in #4(w112) -> ()
    n70 = feedback #5() -> (w124:T1)  [unwired: 1 in]
    n71 = feedback-in #5(w121) -> ()
    n72 = feedback #6() -> (w132:bool)  [unwired: 1 in]
    "packet start" <- w132
    n73 = call "send power.vi"("packet start"=w132, "input valid"=w118, "sample"=w134) -> ()  [unwired: 9 in]
    n74 = Boolean To (0,1)(Boolean=w132) -> (0, 1=w150:i16)
    n75 = To Unsigned Long Integer(number=w150) -> (unsigned 32bit integer=w149:u32)
    n76 = feedback #7() -> (w153:bool)  [unwired: 1 in]
    n77 = call "Synchronization.vi"("channels in"=w121, "use static frequency shift"="use static frequency shift", "input valid"=w112, "primary channel input valid"=w179, "primary channel sample"=w178, "rearm packet detection"=w153) -> ("packet start"=w133:bool, "channels out"=w131:T1, "packet detected"=w155:bool, "sample out valid"=w129:bool, "compensated CFO"=→"compensated CFO":fxp<+/-,48,0>)
    "packet detected" <- w155
    n78 = feedback-in #6(w133) -> ()
    n79 = call "tune samples.vi"("compensation"=w126, "input valid"=w129, "channels in"=w131) -> ("output valid"=w115:bool, "channels out"=w130:T1)  [unwired: 7 in]
    "sample out valid" <- w115
    n80 = Unbundle By Name(w130) -> ("channel 1"=→"sample out":T5)
    n81 = call "send samples.vi"("sample valid before CFO"=w113, "use before CFO"="save before CFO", "channels before CFO"=w124, "packet start"=w132, "sample valid after CFO"=w115, "channels after CFO"=w130) -> ()  [unwired: 6 in]
    n82 = call "RX IQ Processing.vi"("configuration"="configuration", "packet start"=w132, "channels in"=w130, "input valid"=w115) -> ("channel estimate timing"=w148:T30, "channel estimate"=w136:T31, "last sample"=w154:bool, "subcarrier index"=→"subcarrier index":fxp<+/-,9,9>, "output valid"=w145:bool)  [unwired: 4 in, 3 out]
    "channel estimate valid" <- w145
    n83 = feedback-in #7(w154) -> ()
    n84 = feedback #8(u32 0) -> (w170:u32)
    n85 = Add(x=w149, y=w170) -> (x+y=w152:u32)
    "packet start number" <- w152
    n86 = feedback-in #8(w152) -> ()
    n87 = feedback #9(FALSE) -> (w157:bool)
    n88 = case shown="True" w155 {
      tunnel: [w183 TRUE] -> w158
      tunnel: w157 -> [w183 _]
      frame False {
      }
      frame True {
      }
    }
    "was packet detected true? 2" <- w158
    n89 = feedback-in #9(w158) -> ()
    n90 = feedback #10(FALSE) -> (w160:bool)
    n91 = case shown="False" w132 {
      tunnel: [w185 TRUE] -> w161
      tunnel: w160 -> [w185 _]
      frame False {
      }
      frame True {
      }
    }
    "was packet start true?" <- w161
    n92 = feedback-in #10(w161) -> ()
    n93 = Unbundle By Name("configuration") -> ("format"=w146:enum16{"NON_HT_OFDM", "VHT", "NON_HT_DUP_OFDM"})
    n94 = call "Send CSI.vi"("csi valid"=w145, "channel estimate timing"=w148, "channel estimate"=w136, "format"=w146) -> ()  [unwired: 8 in]
    n95 = Unbundle By Name(w136) -> ("subcarrier channel"=→"channel estimate":T2)
  }
  n96 = node-c288(w16) -> ()
  n97 = node-c288(w2) -> ()
